vi "configure frame pulser.vi"(11 "ADsamples.per.frame":dbl) -> (3 "frame pulser task out":refnum<k21>)   [LabVIEW 2012]
doc: "SciScan 1.2 160622"
uses:
  <vilib>/DAQmx/write.llb/DAQmx Write (Counter Ticks 1Chan 1Samp).vi
  <vilib>/DAQmx/create/channels.llb/DAQmx Create Channel (CO-Pulse Generation-Ticks).vi
  <vilib>/DAQmx/configure/timing.llb/DAQmx Timing (Implicit).vi
  <vilib>/DAQmx/miscellaneous.llb/DAQmx Fill In Error Info.vi
  <resource>/objmgr/daqmx.rc
panel:
  in  "s":bool=TRUE
  out "error out":errorcluster
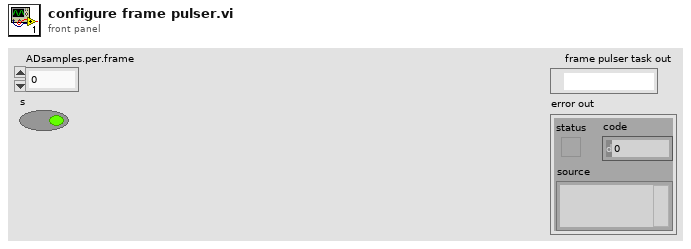
[diagram p1: front panel]
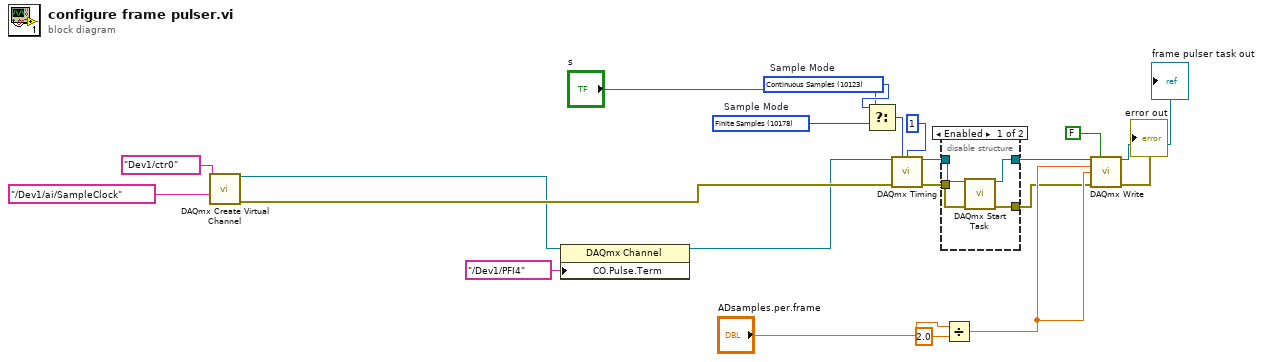
[diagram p0: block diagram]
diagram:
  w6 = 10123 items=["Finite Samples"=10178, "Continuous Samples"=10123, "Hardware Timed Single Point"=12522]  # Sample Mode
  w5 = 10178 items=["Finite Samples"=10178, "Continuous Samples"=10123, "Hardware Timed Single Point"=12522]  # Sample Mode
  n1 = call-poly <vilib>:"DAQmx Create Virtual Channel.vi"("counter"=tag "Dev1/ctr0", "source of ticks"=tag "/Dev1/ai/SampleClock") -> ("task out"=w1:refnum<k21>, "error out"=w19:errorcluster)  [unwired: 12 in]
  n2 = property class="DAQmx Channel"(reference=w1, "CO.Pulse.Term"=tag "/Dev1/PFI4") -> (reference out=w17:refnum<k21>)  [unwired: 1 in, 1 out]
  n3 = Select(t=w6, s="s", f=w5) -> (s? t:f=w7:i32)
  n4 = call-poly <vilib>:"DAQmx Timing.vi"("task/channels in"=w17, "sample mode"=w7, "samples per channel"=1, "error in"=w19) -> ("task out"=w15:refnum<k21>, "error out"=w10:errorcluster)  [unwired: 10 in]
  n5 = disable-structure shown="Enabled" {
    disable-tunnel: w15 -> [w25 w27]
    disable-tunnel: [w24 w27] -> w14
    disable-tunnel: w10 -> [w23 w26]
    disable-tunnel: [w22 w26] -> w9
    frame Enabled {
      n6 = call <vilib>:"DAQmx Start Task.vi"("task/channels in"=w25, "error in"=w23) -> ("task out"=w24:refnum<k21>, "error out"=w22:errorcluster)  [unwired: 12 in]
    }
    frame Disabled {
    }
  }
  n7 = Divide(x="ADsamples.per.frame", y=2.0) -> (x/y=w11:dbl)
  n8 = call-poly <vilib>:"DAQmx Write.vi"("task/channels in"=w14, "auto start"=FALSE, "high ticks"=w11, "low ticks"=w11, "error in"=w9) -> ("task out"=→"frame pulser task out":refnum<k21>, "error out"=→"error out":errorcluster)  [unwired: 8 in, 1 out]
